vi "Create Instrument.vi"(8 "error in":errorcluster, 10 "Instrument Identifier":string) -> (0 "error out":errorcluster, 2 "IInstrument out":refnum<class "IInstrument.lvclass">)   [LabVIEW 2024, in "Instrument Manager.lvclass"]
uses:
  Instrument Manager.lvclass
  Interfaces/IInstrument/IInstrument.lvclass
  Interfaces/IUnmanaged/IUnmanaged.lvclass
  Interfaces/IConfigure/IConfigure.lvclass
  Interfaces/IConfigurable/IConfigurable.lvclass
  Config from JSON/Config from JSON.lvclass
  D:/git/HAL/Source/Interfaces/IConfiguration/IConfiguration.lvclass
  Instrument Manager.lvclass/Instrument Manager.ctl
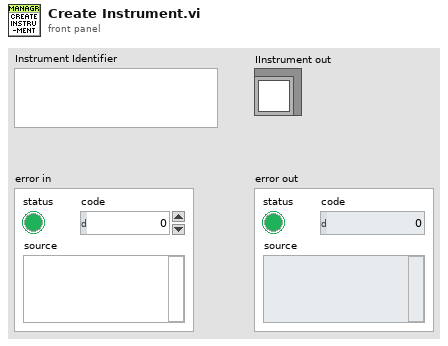
[diagram p1: front panel]
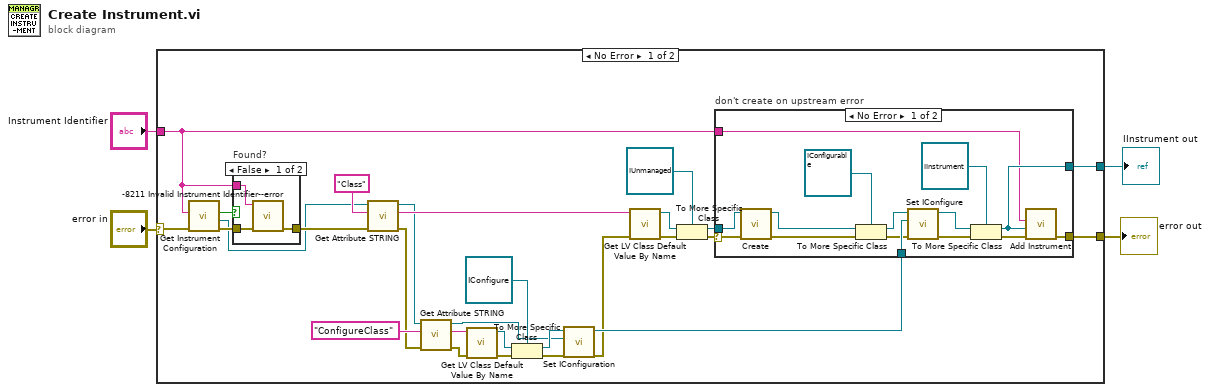
[diagram p0: block diagram]
diagram:
  n1 = case shown="No Error" "error in" {
    selector: "error in" -> [w31 w52]
    tunnel: [w30 w52] -> w3
    tunnel: "Instrument Identifier" -> [w28 _]
    tunnel: [w29 _] -> w1
    frame No Error {
      n2 = call "Get Instrument Configuration.vi"("Error In"=w31, "Instrument Identifier"=w28) -> ("Error Out"=w9:errorcluster, "Instrument Configuration"=w5:refnum<class "Config from JSON.lvclass">, "Found"=w10:bool)  [unwired: 7 in]
      n3 = case "Found?" shown="False" w10 {
        tunnel: w9 -> [w50 w51]
        tunnel: [w49 w51] -> w8
        tunnel: w28 -> [w48 _]
        frame False {
          n4 = call "-8211 Invalid Instrument Identifier--error.vi"("error in"=w50, "Source"=w48) -> ("error out"=w49:errorcluster)  [unwired: 9 in]
        }
        frame True {
        }
      }
      n5 = call-dynamic "Get Attribute STRING.vi"("error in"=w8, "Attribute"="Class", "ConfigFromJSON in"=w5) -> ("error out"=w14:errorcluster, "Value"=w26:string, "ConfigFromJSON out"=w16:refnum<class "Config from JSON.lvclass">)  [unwired: 6 in]
      n6 = call-dynamic "Get Attribute STRING.vi"("error in"=w14, "Attribute"="ConfigureClass", "ConfigFromJSON in"=w16) -> ("error out"=w21:errorcluster, "Value"=w22:string, "ConfigFromJSON out"=w11:refnum<class "Config from JSON.lvclass">)  [unwired: 6 in]
      n7 = call <vilib>:"Get LV Class Default Value By Name.vi"("error in (no error)"=w21, "class name"=w22) -> ("error out"=w20:errorcluster, "object"=w19:refnum<class>)  [unwired: 8 in]
      n8 = To More Specific Class(target class=refnum<class "IConfigure.lvclass"> refnum ("IConfigure.lvclass"), reference=w19, error in=w20) -> (specific class reference=w17:refnum<class "IConfigure.lvclass">, error out=w13:errorcluster)
      n9 = call-dynamic "Set IConfiguration.vi"("IConfiguration"=w11, "IConfigure in"=w17) -> ("IConfigure out"=w15:refnum<class "IConfigure.lvclass">)  [unwired: 9 in]
      n10 = call <vilib>:"Get LV Class Default Value By Name.vi"("error in (no error)"=w13, "class name"=w26) -> ("error out"=w24:errorcluster, "object"=w25:refnum<class>)  [unwired: 8 in]
      n11 = To More Specific Class(target class=refnum<class "IUnmanaged.lvclass"> refnum ("IUnmanaged.lvclass"), reference=w25, error in=w24) -> (specific class reference=w6:refnum<class "IUnmanaged.lvclass">, error out=w7:errorcluster)
      n12 = case "don't create on upstream error" shown="No Error" w7 {
        selector: w7 -> [w38 w47]
        tunnel: w15 -> [w45 _]
        tunnel: [w42 w47] -> w30
        tunnel: [w41 _] -> w29
        tunnel: w28 -> [w40 _]
        tunnel: w6 -> [w33 _]
        frame No Error {
          n13 = call-dynamic "Create.vi"("error in"=w38, "IUnmanaged in"=w33) -> ("error out"=w34:errorcluster, "IUnmanaged out"=w32:refnum<class "IUnmanaged.lvclass">)  [unwired: 8 in]
          n14 = To More Specific Class(target class=refnum<class "IConfigurable.lvclass"> refnum ("IConfigurable.lvclass"), reference=w32, error in=w34) -> (specific class reference=w36:refnum<class "IConfigurable.lvclass">, error out=w37:errorcluster)
          n15 = call-dynamic "Set IConfigure.vi"("error in"=w37, "IConfigure"=w45, "IConfigurable in"=w36) -> ("error out"=w39:errorcluster, "IConfigurable out"=w46:refnum<class "IConfigurable.lvclass">)  [unwired: 7 in]
          n16 = To More Specific Class(target class=refnum<class "IInstrument.lvclass"> refnum ("IInstrument.lvclass"), reference=w46, error in=w39) -> (specific class reference=w41:refnum<class "IInstrument.lvclass">, error out=w43:errorcluster)
          n17 = call "Add Instrument.vi"("Error In"=w43, "IInstrument"=w41, "Instrument Identifier"=w40) -> ("Error Out"=w42:errorcluster)  [unwired: 8 in]
        }
        frame Error {
        }
      }
    }
    frame Error {
    }
  }
  "error out" <- w3
  "IInstrument out" <- w1
